vi "TCP_Server_Test.vi"() -> ()   [LabVIEW 2020]
doc: "Demonstrates how to set up a basic TCP connection, send data to the specified port once a connection has been established, and terminate the connection once the data has been sent. This VI is designed to stop if the TCP connection is terminated. The data sent in this example is an array of random numbers."
panel:
  out "Read":string
  in  "Send":bool
  in  "Send":string
  in  "Client Closed":string="The client VI closed the connection."
  in  "Stop":bool
  # "Overview: Demonstrates the use of the TCP functions to initialize a TCP server that can send data to a client VI.\nInstructions:\n1. Run the VI.\n2. Open Simple TCP - Client.vi and follow the instructions on its front panel. Note that if you wait longer than 30 seconds to do this after running this VI, it will time out.\n3. Click Stop to stop the VI. Note that if you stop the client VI, this VI will stop automatically."
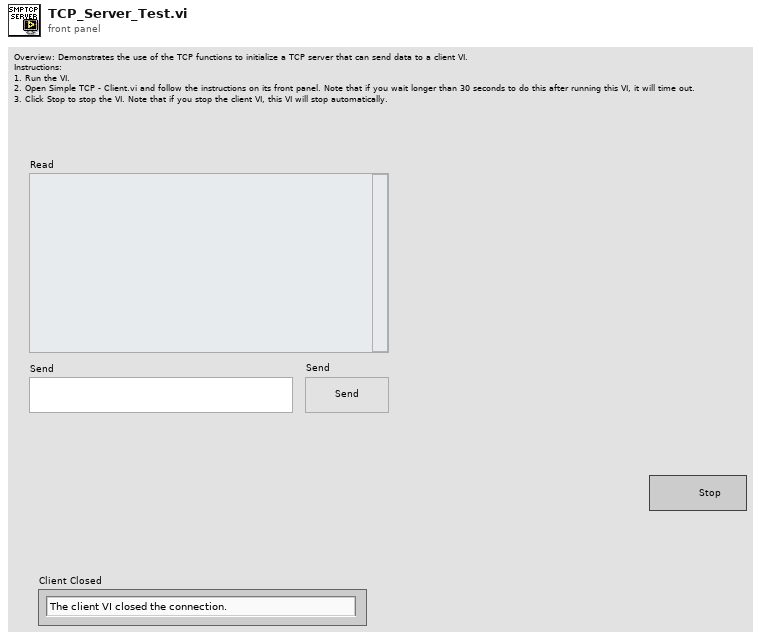
[diagram p1: front panel]
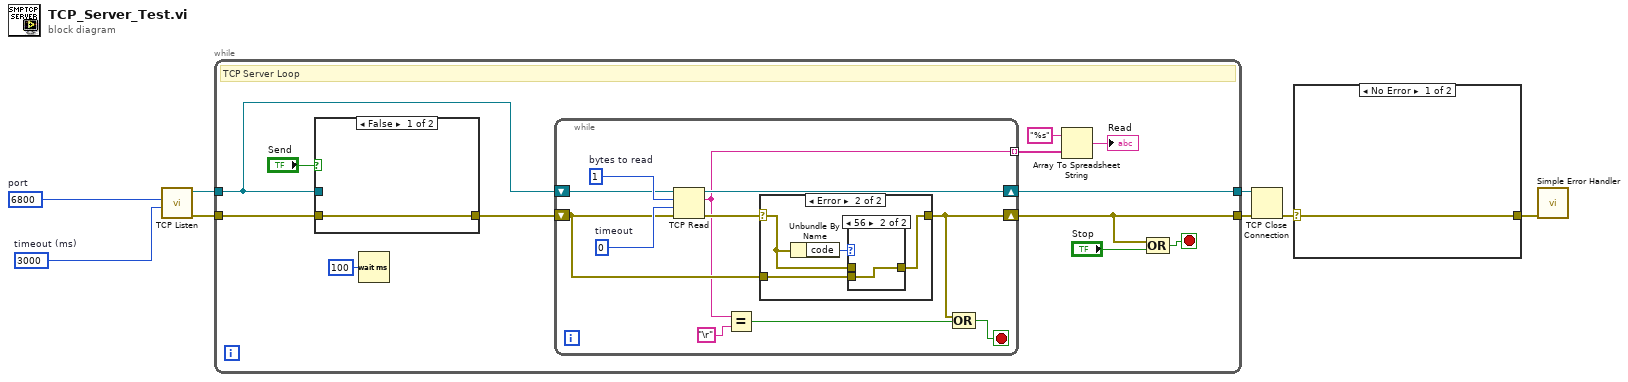
[diagram p0: block diagram]
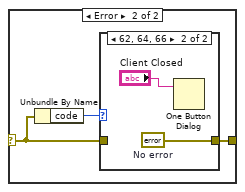
[diagram p2: hidden frame]
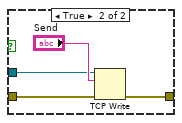
[diagram p6: hidden frame]
diagram:
  w1 = u16 6800  # port
  w2 = 3000  # timeout (ms)
  n1 = call <vilib>:"TCP Listen.vi"("timeout ms (wait forever: -1)"=w2, "port"=w1) -> ("error out"=w3:errorcluster, "connection ID"=w4:refnum<k5>)  [unwired: 5 in, 3 out]
  n2 = while {
    tunnel: [w16] -> w7
    tunnel: [w17] -> w8
    tunnel: w4 -> [w12]
    tunnel: w3 -> [w14]
    stop <- w19 stop-if-true
    # "TCP Server Loop"
    n3 = case shown="False" "Send" {
      tunnel: [w39 w43] -> w15
      tunnel: w14 -> [w39 w42]
      tunnel: w12 -> [_ w40]
      frame False {
      }
      frame True {
        n4 = TCP Write(connection ID=w40, data in="Send", error in (no error)=w42) -> (error out=w43:errorcluster)  [unwired: 3 out]
      }
    }
    n5 = Wait (ms)(milliseconds to wait=u32 100) -> ()  [unwired: 1 out]
    n6 = while {
      shift-right: [w22] -> w16
      shift-left: w15 -> [w27]
      shift-right: [w30] -> w17
      shift-left: w12 -> [w26]
      tunnel: [w21] -> w11 mode=indexing
      stop <- w23 stop-if-true
      w29 = 0  # timeout
      w31 = 1  # bytes to read
      n7 = TCP Read(connection ID=w26, bytes to read=w31, error in (no error)=w27, 9:w29) -> (connection ID out=w30:refnum<k5>, data out=w21:string, error out=w28:errorcluster)  [unwired: 1 out]
      n8 = Equal?(x=w21, y="\r") -> (x = y?=w24:bool)
      n9 = case shown="Error" w28 {
        selector: w28 -> [w32 w35]
        tunnel: [w32 w33] -> w22
        tunnel: w27 -> [_ w34]
        frame No Error {
        }
        frame Error {
          n10 = Unbundle By Name(w35) -> ("code"=w36:i32)
          n11 = case shown="56" w36 {
            tunnel: w35 -> [w37 _]
            tunnel: w34 -> [_ w38]
            tunnel: [w37 w38] -> w33
            frame Default {
            }
            frame 56 {
            }
          }
        }
      }
      n12 = Compound Arithmetic op=OR(w22, w24) -> (w23:bool)
    }
    n13 = Array To Spreadsheet String(array=w11, 3:"%s" ("format string")) -> (spreadsheet string=→"Read":string)  [unwired: 1 in]
    n14 = Compound Arithmetic op=OR(w16, "Stop") -> (w19:bool)
  }
  n15 = TCP Close Connection(connection ID=w8, error in (no error)=w7) -> (error out=w6:errorcluster)  [unwired: 2 out]
  n16 = case shown="No Error" w6 {
    selector: w6 -> [w44 w46]
    tunnel: [w44 w45] -> w5
    frame No Error {
    }
    frame Error {
      n17 = Unbundle By Name(w46) -> ("code"=w47:i32)
      n18 = case shown="62, 64, 66" w47 {
        tunnel: w46 -> [w48 _]
        tunnel: [w48 w50] -> w45
        frame Default {
        }
        frame 62, 64, 66 {
          w50 = errorcluster {"status"=FALSE, "code"=0, "source"=""}  # No error
          n19 = One Button Dialog(message="Client Closed") -> ()  [unwired: 1 in, 1 out]
        }
      }
    }
  }
  n20 = call <vilib>:"Simple Error Handler.vi"("error in (no error)"=w5) -> ()  [unwired: 1 in, 8 out]
